vi "conv_Cernox_R2T.vi"(6 "data_in":dbl[][](array[numeric]), 7 "Cernox ID":enum16{"X130217"}(ring), 8 "error in":errorcluster, 11 "R":dbl=40.0) -> (0 "error out":errorcluster, 3 "T":dbl, 4 "data_out":dbl[][](array[numeric]))   [LabVIEW 2019]
uses:
  <vilib>/Utility/file.llb/Read Delimited Spreadsheet (DBL).vi
panel:
  out "X":dbl
  out "Z":dbl
  out "Z_U":dbl
  out "Z_L":dbl
  out "R_U":dbl
  out "R_L":dbl
  out "index":i32
  out "array_coef":dbl[](array[numeric])
  # "VI to convert Cernox resistance to temperature.\n\ndata_out can/should be fed back to data_in \nso as to read the data file only once."
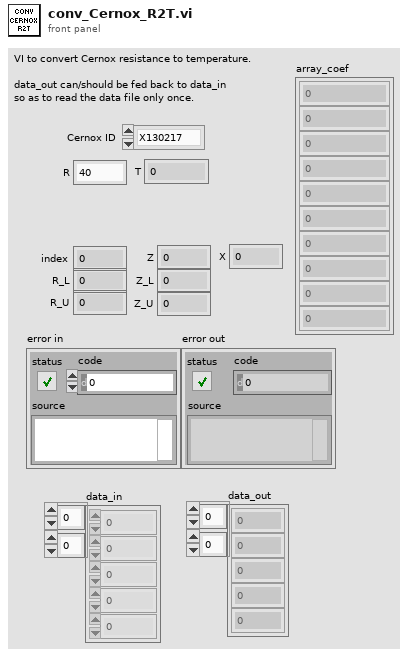
[diagram p1: front panel]
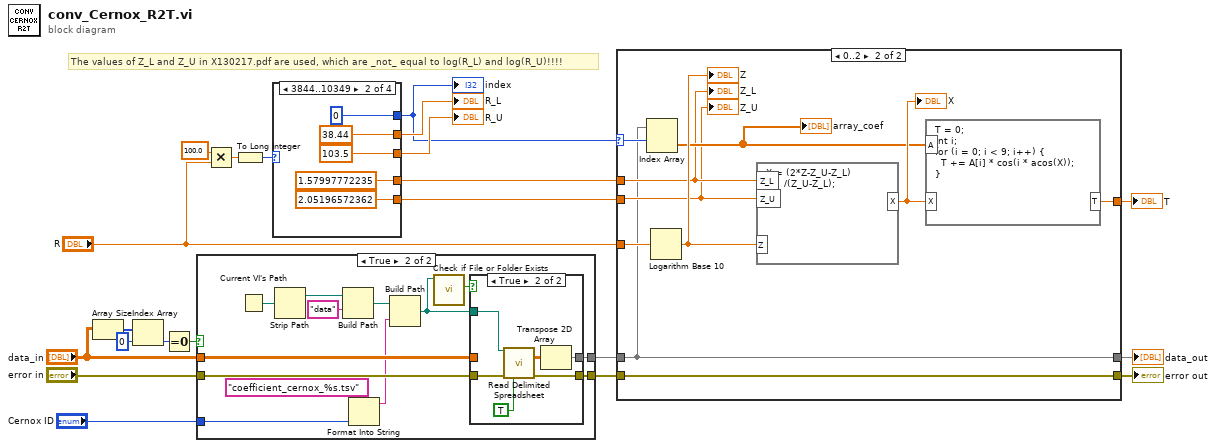
[diagram p0: block diagram]
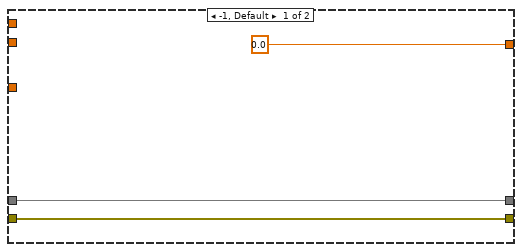
[diagram p2: hidden frame]
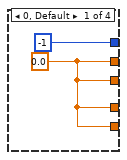
[diagram p3: hidden frame]
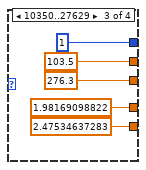
[diagram p4: hidden frame]
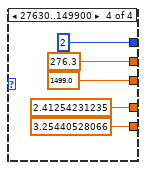
[diagram p5: hidden frame]
diagram:
  # "The values of Z_L and Z_U in X130217.pdf are used, which are _not_ equal to log(R_L) and log(R_U)!!!!"
  n1 = Array Size(array="data_in") -> (size(s)=w16:i32[])
  n2 = Index Array(array=w16, index=0) -> (element=w15:i32)
  n3 = Equal To 0?(x=w15) -> (x = 0?=w18:bool)
  n4 = case shown="True" w18 {
    tunnel: "error in" -> [w22 w30]
    tunnel: [w22 w29] -> w20
    tunnel: [w23 w28] -> w17
    tunnel: "data_in" -> [w23 w27]
    tunnel: "Cernox ID" -> [_ w25]
    frame False {
    }
    frame True {
      n5 = Current VI's Path() -> (path=w36:path)
      n6 = Strip Path(path=w36) -> (stripped path=w35:path)  [unwired: 1 out]
      n7 = Build Path(base path=w35, name or relative path="data") -> (appended path=w33:path)
      n8 = Format Into String(format string="coefficient_cernox_%s.tsv" ("name or relative path"), w25) -> (resulting string=w24:string)  [unwired: 2 in, 1 out]
      n9 = Build Path(base path=w33, name or relative path=w24) -> (appended path=w31:path)
      n10 = call <vilib>:"Check if File or Folder Exists.vi"("path"=w31) -> ("file or folder exists?"=w32:bool)  [unwired: 8 in, 2 out]
      n11 = case shown="True" w32 {
        tunnel: w31 -> [_ w44]
        tunnel: w30 -> [w37 w43]
        tunnel: [w37 w42] -> w29
        tunnel: [w38 w39] -> w28
        tunnel: w27 -> [w38 _]
        frame False {
        }
        frame True {
          n12 = call-poly <vilib>:"Read Delimited Spreadsheet.vi"("file path (dialog if empty)"=w44, "error in (no error)"=w43, "transpose? (F)"=TRUE) -> ("all rows"=w40:dbl[][], "error out"=w42:errorcluster)  [unwired: 7 in, 4 out]
          n13 = Transpose 2D Array(2D array=w40) -> (transposed array=w39:dbl[][])
        }
      }
    }
  }
  n14 = Multiply(x=100.0, y="R") -> (x*y=w11:dbl)
  n15 = To Long Integer(number=w11) -> (32bit integer=w10:i32)
  n16 = case shown="3844..10349" w10 {
    tunnel: [-1 0 1 2] -> w3
    tunnel: [w45 38.44 103.5 276.3] -> w9
    tunnel: [w45 103.5 276.3 1499.0] -> w8
    tunnel: [w45 1.57997772235 1.98169098822 2.41254231235] -> w5
    tunnel: [w45 2.05196572362 2.47534637283 3.25440528066] -> w4
    frame 0, Default {
      w45 = 0.0
    }
    frame 3844..10349 {
    }
    frame 10350..27629 {
    }
    frame 27630..149900 {
    }
  }
  "index" <- w3
  "R_L" <- w9
  "R_U" <- w8
  n17 = case shown="0..2" w3 {
    selector: w3 -> [_ w72]
    tunnel: w20 -> [w62 w65]
    tunnel: w17 -> [w63 w66]
    tunnel: w5 -> [_ w68]
    tunnel: "R" -> [_ w74]
    tunnel: [0.0 w69] -> w6
    tunnel: w4 -> [_ w67]
    tunnel: [w63 w66] -> w2
    tunnel: [w62 w65] -> w1
    frame -1, Default {
    }
    frame 0..2 {
      n18 = Index Array(array=w66, index (row)=w72) -> (element=w70:dbl[])  [unwired: 1 in]
      "array_coef" <- w70
      n19 = Logarithm Base 10(1:w74) -> (0:w73:dbl)
      "Z" <- w73
      n20 = formula code="X = (2*Z-Z_U-Z_L)\n      /(Z_U-Z_L);"("Z"=w73, "Z_U"=w67, "Z_L"=w68) -> ("X"=w71:dbl)
      "X" <- w71
      n21 = formula code="T = 0;\nint i;\nfor (i = 0; i < 9; i++) {\n  T += A[i] * cos(i * acos(X));\n}"("X"=w71, "A"=w70) -> ("T"=w69:dbl)
      "Z_L" <- w68
      "Z_U" <- w67
    }
  }
  "T" <- w6
  "data_out" <- w2
  "error out" <- w1
